vi "HatchInOpen.vi"(8 "error in (no error)":errorcluster, 11 "HatchIn in":refnum<class "HatchIn.lvclass">) -> (0 "error out":errorcluster, 3 "HatchIn out":refnum<class "HatchIn.lvclass">)   [LabVIEW 2018, in "HatchIn.lvclass"]
uses:
  HatchIn.lvclass
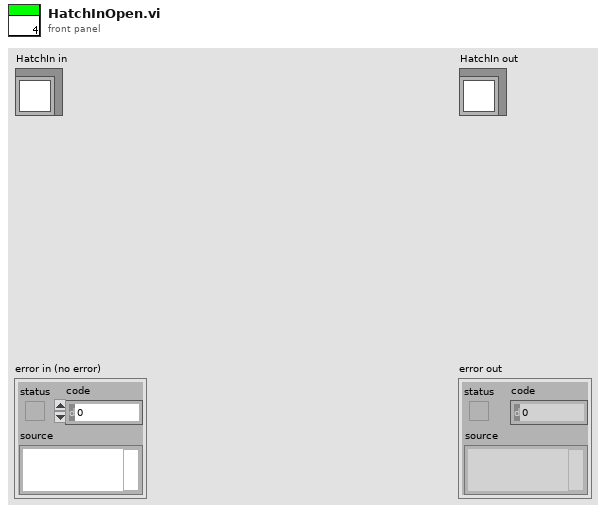
[diagram p1: front panel]
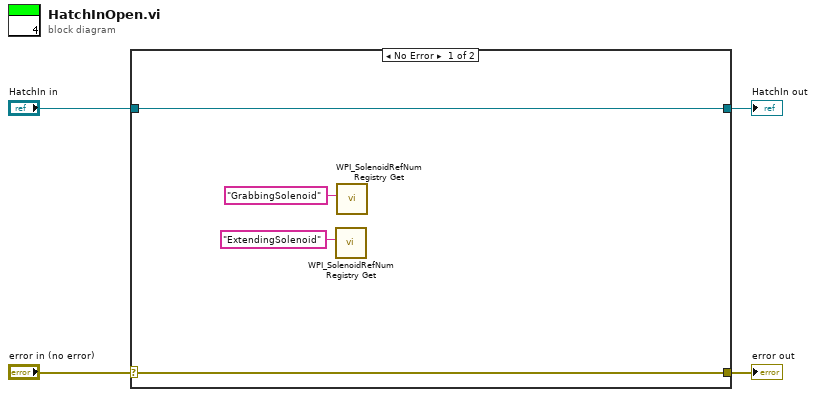
[diagram p0: block diagram]
diagram:
  n1 = case shown="No Error" "error in (no error)" {
    selector: "error in (no error)" -> [w7 w10]
    tunnel: [w7 w10] -> w3
    tunnel: [w8 w9] -> w1
    tunnel: "HatchIn in" -> [w8 w9]
    frame No Error {
      n2 = call <vilib>:"WPI_SolenoidRefNum Registry Get.vi"("refnum name"="ExtendingSolenoid") -> ()  [unwired: 9 in, 2 out]
      n3 = call <vilib>:"WPI_SolenoidRefNum Registry Get.vi"("refnum name"="GrabbingSolenoid") -> ()  [unwired: 9 in, 2 out]
    }
    frame Error {
    }
  }
  "error out" <- w3
  "HatchIn out" <- w1
